vi "SW_Gen_Check_segments_parameters.vi"(3 "Image plotting parameters":T1) -> (1 "Corrected image plotting parameters":T1)   [LabVIEW 2018, in "Tracker.lvlib"]
uses:
  Tracker.lvlib
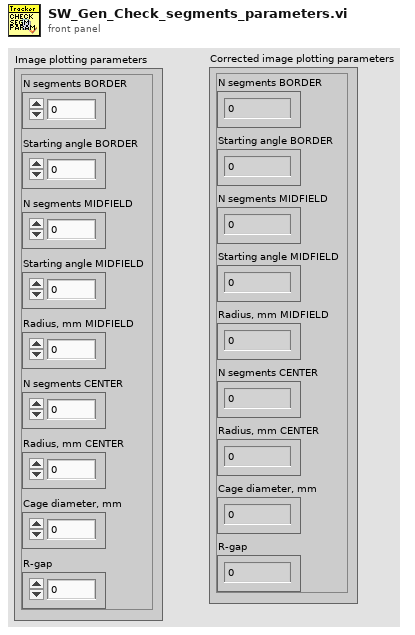
[diagram p1: front panel]
types:
  T1 = cluster{"N segments BORDER":u8, "Starting angle BORDER":i16, "N segments MIDFIELD":u8, "Starting angle MIDFIELD":i16, "Radius, mm MIDFIELD":u16, "N segments CENTER":u8, "Radius, mm CENTER":u16, "Cage diameter, mm":u16, "R-gap":i32}
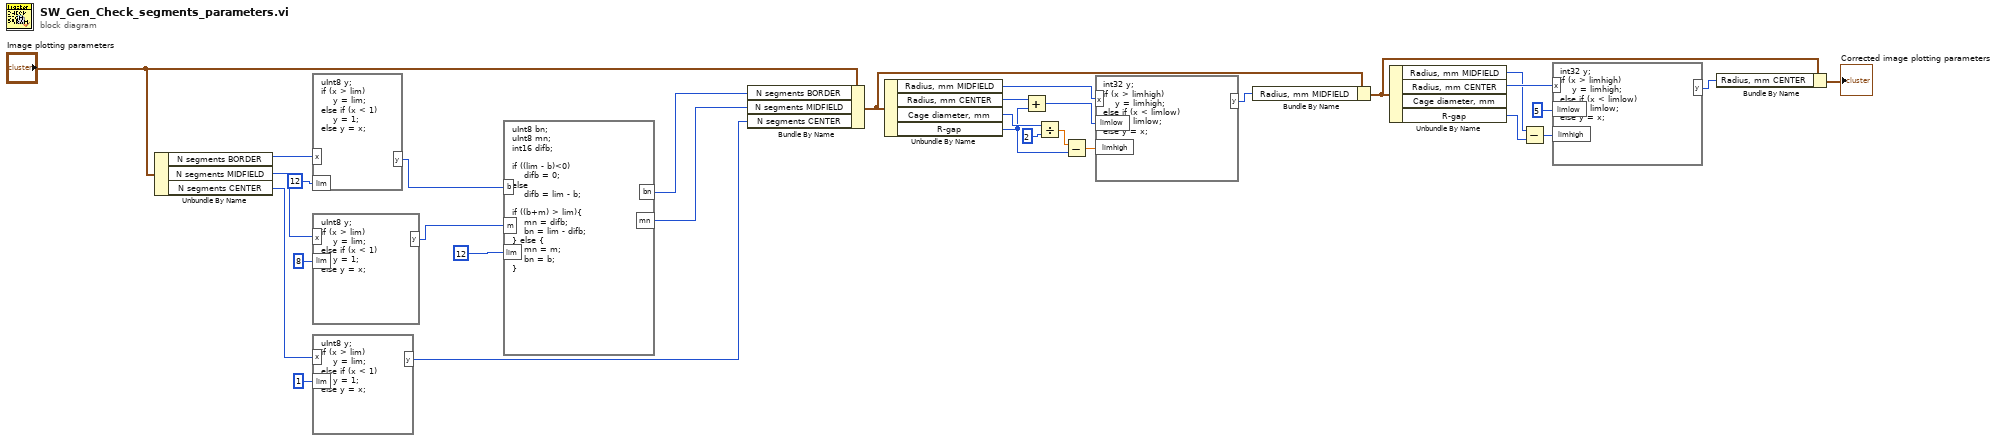
[diagram p0: block diagram]
diagram:
  n1 = Unbundle By Name("Image plotting parameters") -> ("N segments BORDER"=w31:u8, "N segments MIDFIELD"=w30:u8, "N segments CENTER"=w29:u8)
  n2 = formula code="uInt8 y;\nif (x > lim)\n    y = lim;\nelse if (x < 1)\n    y = 1;\nelse y = x;"("x"=w31, "lim"=u8 12 ("input variable")) -> ("y"=w5:u8)
  n3 = formula code="uInt8 y;\nif (x > lim)\n    y = lim;\nelse if (x < 1)\n    y = 1;\nelse y = x;"("x"=w30, "lim"=u8 8 ("input variable")) -> ("y"=w4:u8)
  n4 = formula code="uInt8 y;\nif (x > lim)\n    y = lim;\nelse if (x < 1)\n    y = 1;\nelse y = x;"("x"=w29, "lim"=u8 1 ("input variable")) -> ("y"=w25:u8)
  n5 = formula code="uInt8 bn;\nuInt8 mn;\nint16 difb;\n\nif ((lim - b)<0) \n    difb = 0;\nelse\n    difb = lim - b;\n\nif ((b+m) > lim){\n    mn = difb;\n    bn = lim - difb;\n} else {\n    mn = m;\n    bn = b;\n}"("b"=w5, "m"=w4, "lim"=u8 12 ("input variable")) -> ("bn"=w3:u8, "mn"=w2:u8)
  n6 = Bundle By Name(cluster="Image plotting parameters", "N segments BORDER"=w3, "N segments MIDFIELD"=w2, "N segments CENTER"=w25) -> (w6:T1)
  n7 = Unbundle By Name(w6) -> ("Radius, mm MIDFIELD"=w24:u16, "Radius, mm CENTER"=w19:u16, "Cage diameter, mm"=w23:u16, "R-gap"=w18:i32)
  n8 = Add(x=w19, y=w18) -> (x+y=w17:i32)
  n9 = Divide(x=w23, y=u16 2) -> (x/y=w21:dbl)
  n10 = Subtract(x=w21, y=w18) -> (x-y=w20:dbl)
  n11 = formula code="int32 y;\nif (x > limhigh)\n    y = limhigh;\nelse if (x < limlow)\n    y = limlow;\nelse y = x;"("x"=w24, "limlow"=w17, "limhigh"=w20) -> ("y"=w16:i32)
  n12 = Bundle By Name(cluster=w6, "Radius, mm MIDFIELD"=w16) -> (w10:T1)
  n13 = Unbundle By Name(w10) -> ("Radius, mm MIDFIELD"=w13:u16, "Radius, mm CENTER"=w15:u16, "R-gap"=w12:i32)  [unwired: 1 out]
  n14 = Subtract(x=w13, y=w12) -> (x-y=w11:i32)
  n15 = formula code="int32 y;\nif (x > limhigh)\n    y = limhigh;\nelse if (x < limlow)\n    y = limlow;\nelse y = x;"("x"=w15, "limlow"=5 ("input variable"), "limhigh"=w11) -> ("y"=w9:i32)
  n16 = Bundle By Name(cluster=w10, "Radius, mm CENTER"=w9) -> (→"Corrected image plotting parameters":T1)
